vi "get_featurestudio_features.vi"(0 "Device In":T1, 5 "did":string, 7 "wid":string, 9 "eid":string, 11 "error in":errorcluster) -> (4 "Device Oout":T1, 15 "error out":errorcluster)   [LabVIEW 2019]
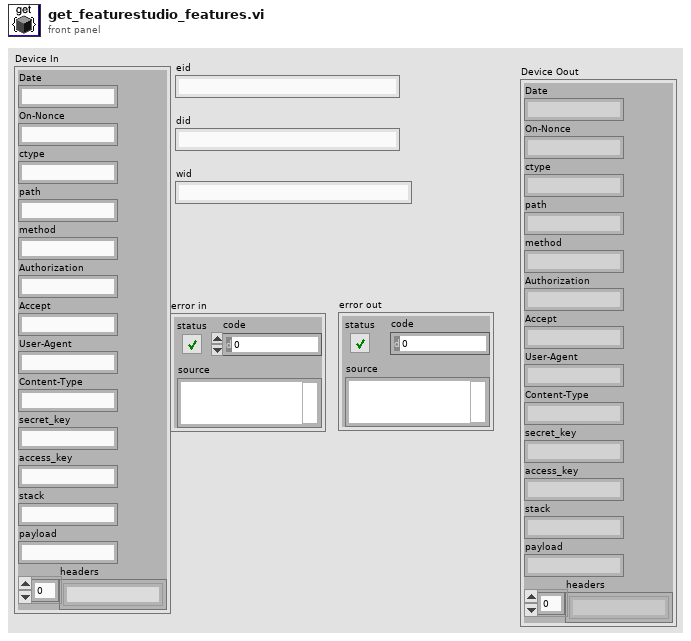
[diagram p1: front panel]
types:
  T1 = cluster{"Date":string, "On-Nonce":string, "ctype":string, "path":string, "method":string, "Authorization":string, "Accept":string, "User-Agent":string, "Content-Type":string, "secret_key":string, "access_key":string, "stack":string, "payload":string, "headers":string[]}
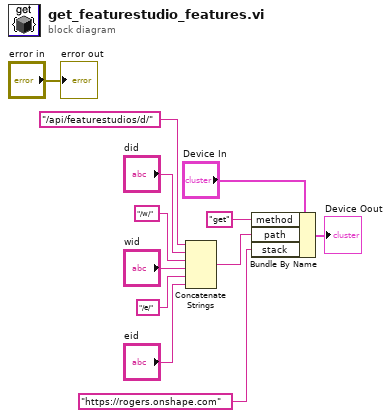
[diagram p0: block diagram]
diagram:
  n1 = Concatenate Strings("/api/featurestudios/d/" ("payload"), "did", "/w/" ("string"), "wid", "/e/" ("string"), "eid") -> (w3:string)
  n2 = Bundle By Name(cluster="Device In", "method"="get" ("Method"), "path"=w3, "stack"="https://rogers.onshape.com" ("stacks")) -> (→"Device Oout":T1)
  "error out" <- "error in"
